vi "测量流程.vi"(11 "控制命令":T1(ring)) -> ()   [LabVIEW 2016, in "斯坦道氨氮V2.lvlib"]
panel:
  out "x-y":dbl
  out "当前时间":timestamp
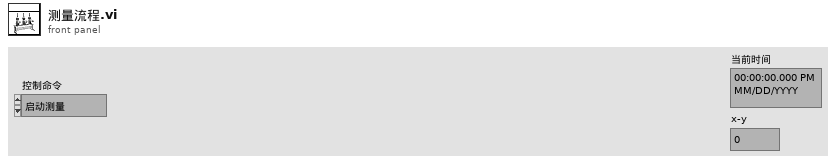
[diagram p1: front panel]
types:
  T1 = enum16{"启动测量", "标样核查", "零点核查", "跨度核查", "空白测试", "平行样测试", "加标回收", "空白校准", "标样校准", "初始化（清洗）", "停止测试", "仪器重启", "校时", "模式设置", "测量间隔设置"}
  T2 = cluster{"站号":u16, "量程切换":enum32{"H", "L", "AUTO"}, "控制命令":enum16{"启动测量", "标样核查", "零点核查", "跨度核查", "空白测试", "平行样测试", "加标回收", "空白校准", "标样校准", "初始化（清洗）", "停止测试", "仪器重启", "校时", "模式设置", "测量间隔设置"}, "模式设置":enum16{"待机", "连续模式", "周期模式", "定点模式", "受控模式", "手动模式"}, "测量间隔":u16}
  T3 = cluster{"时间标识":timestamp, "设备":string, "日志信息":string, "流程参数":string}
  T4 = enum16{"空闲", "水样测试", "标样核查", "零点核查", "跨度核查", "空白测试", "平行样测试", "加标回收", "空白校准", "标样校准", "初始化（清洗）"}
  T5 = cluster{"系统时间":timestamp, "工作状态":u16, "测量模式":enum16{"待机", "连续模式", "周期模式", "定点模式", "受控模式", "手动模式"}, "告警代码":u16, "故障代码":u16, "日志代码":u16, "软件版本":u16, "F0":sgl, "F1":sgl, "F2":sgl, "F3":sgl, "T":sgl, "H":sgl, "id":u16, "flowid":u16, "量程":u16, "总磷控温温度1":sgl, "营养盐控温温度2":sgl, "ADC":sgl}
  T6 = cluster{"水样测试量程模式":enum16{"H", "L", "AUTO"}, "空白核查量程模式":enum16{"H", "L", "AUTO"}, "跨度核查量程模式":enum16{"H", "L", "AUTO"}, "加标回收量程模式":enum16{"H", "L", "AUTO"}, "标样核查量程模式":enum16{"H", "L", "AUTO"}}
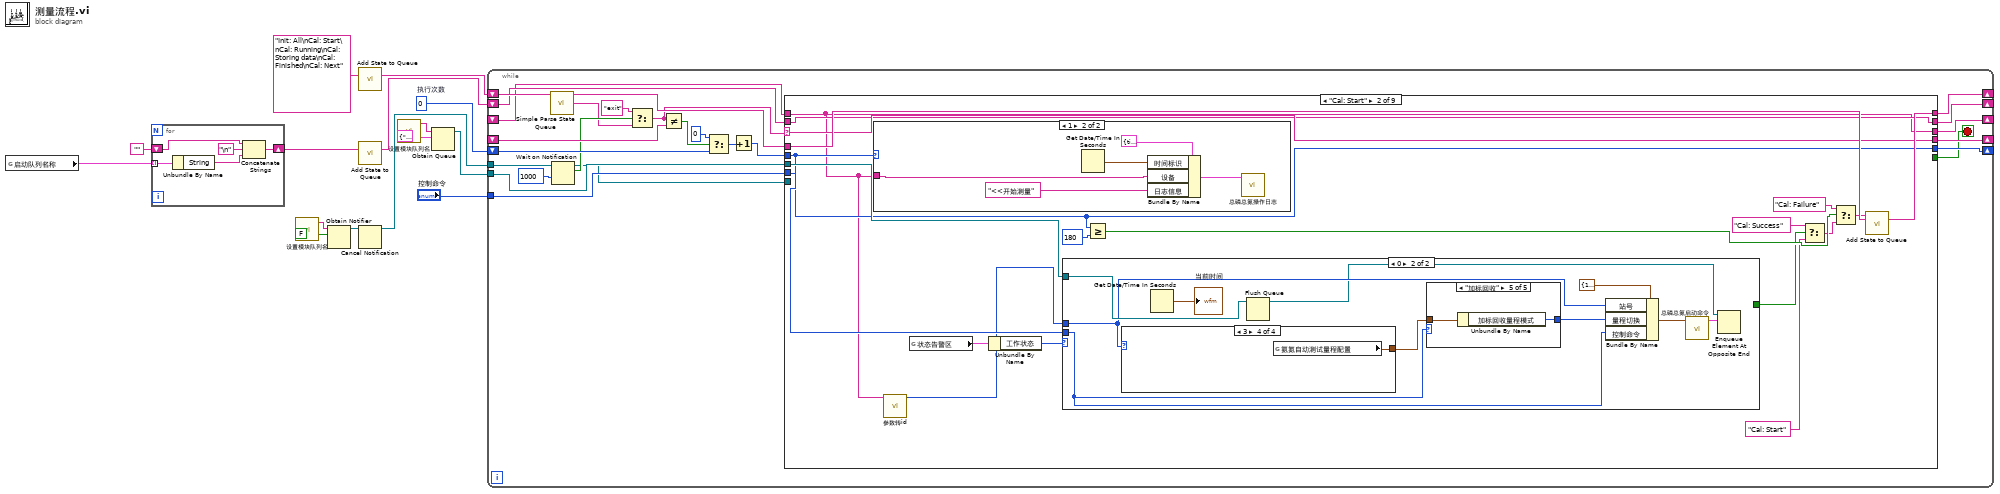
[diagram p0: block diagram]
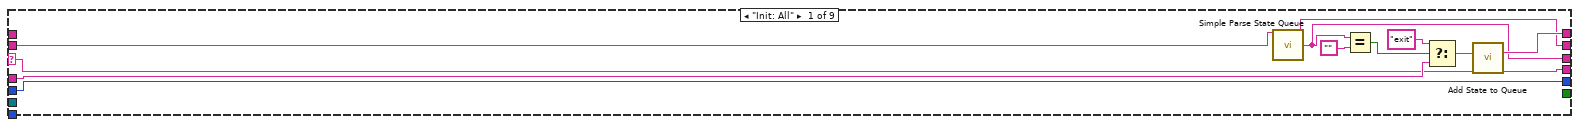
[diagram p2: hidden frame]
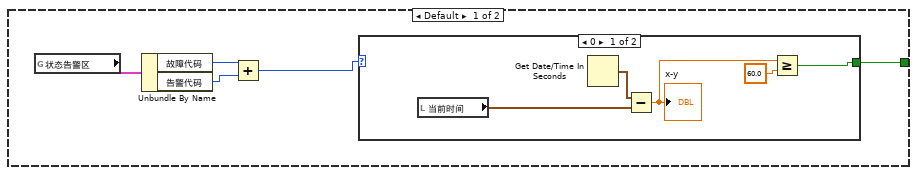
[diagram p3: hidden frame]
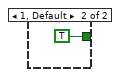
[diagram p4: hidden frame]
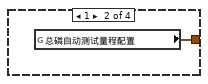
[diagram p6: hidden frame]
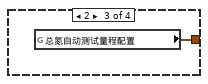
[diagram p7: hidden frame]
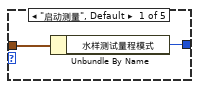
[diagram p8: hidden frame]
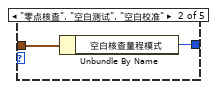
[diagram p9: hidden frame]
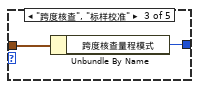
[diagram p10: hidden frame]
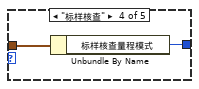
[diagram p11: hidden frame]
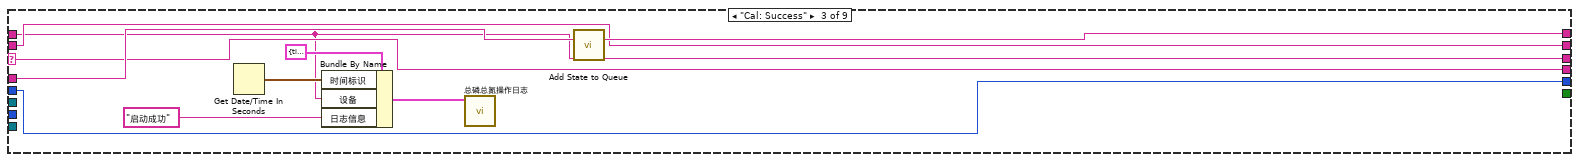
[diagram p13: hidden frame]
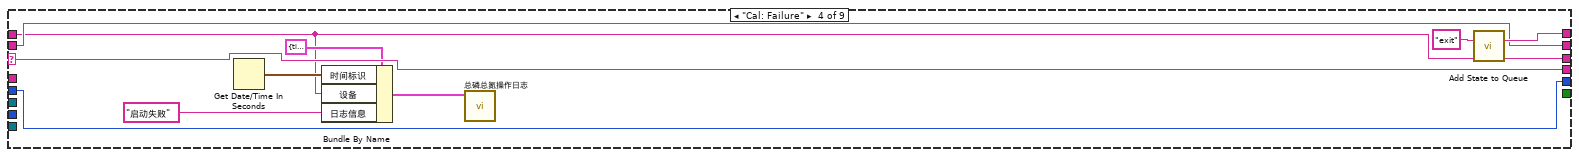
[diagram p14: hidden frame]
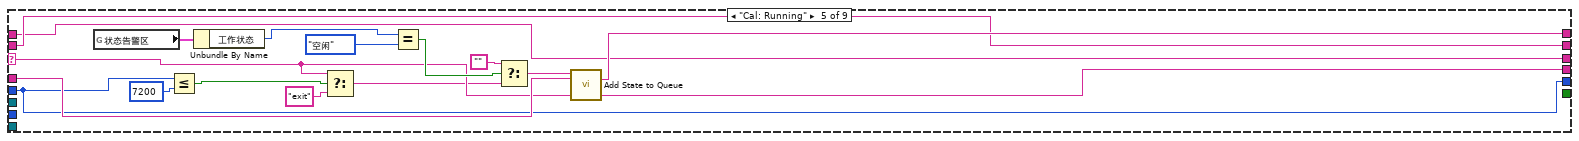
[diagram p15: hidden frame]
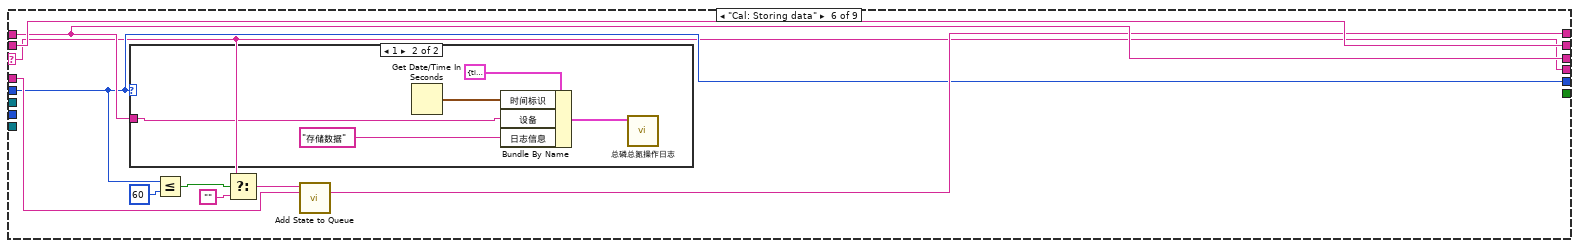
[diagram p16: hidden frame]
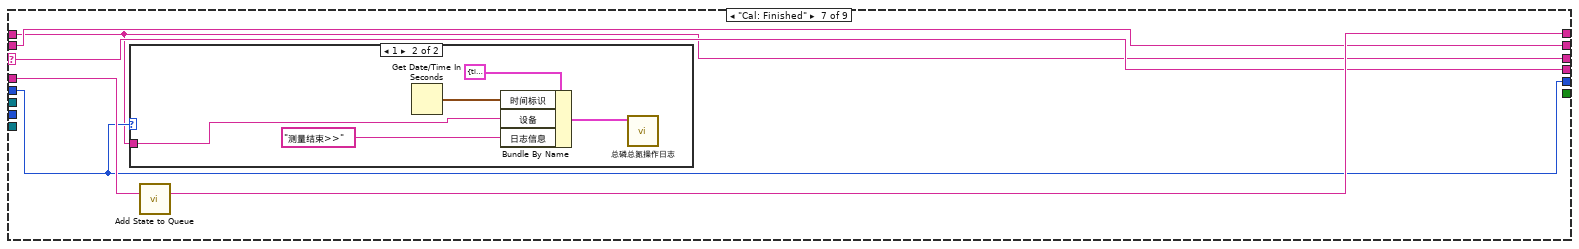
[diagram p18: hidden frame]
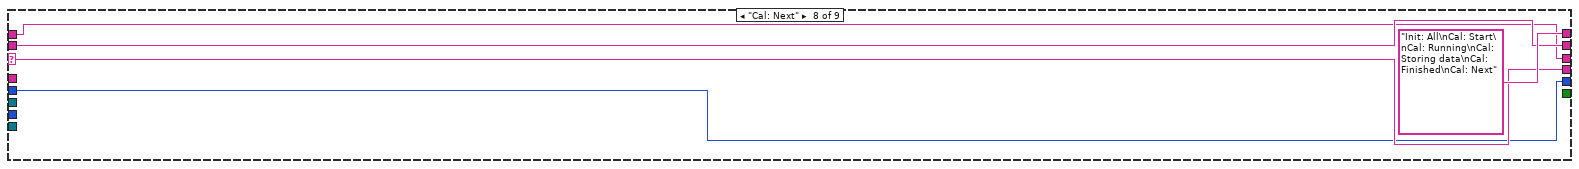
[diagram p20: hidden frame]
diagram:
  w9 = 0  # 执行次数
  n1 = global read "总磷总氮断电保存全局变量.vi" "启动队列名称"() -> (w1:cluster{"String":string, "Value":u16}[])
  n2 = for {
    shift-right: [w19] -> w2
    shift-left: "" -> [w20]
    tunnel: w1 -> [w18] mode=indexing
    n3 = Unbundle By Name(w18) -> ("String"=w17:string)
    n4 = Concatenate Strings(w20, "\n", w17) -> (w19:string)
  }
  n5 = call "设置模块队列名.vi"() -> ("Msg"=w6:string)  [unwired: 5 in]
  n6 = Obtain Notifier(name (unnamed)=w6, notification data type=FALSE) -> (notifier out=w14:refnum<notifier>)  [unwired: 2 in, 2 out]
  n7 = call "Add State to Queue.vi"("State(s) In (\"\")"="Init: All\nCal: Start\nCal: Running\nCal: Storing data\nCal: Finished\nCal: Next" ("State(s) In (\"\")")) -> ("States Out"=w12:string)  [unwired: 14 in]
  n8 = call "Add State to Queue.vi"("State(s) In (\"\")"=w2) -> ("States Out"=w7:string)  [unwired: 14 in]
  n9 = Cancel Notification(0:w14) -> (8:w4:refnum<notifier>)  [unwired: 1 in, 2 out]
  n10 = call "设置模块队列名.vi"() -> ("Msg"=w5:string)  [unwired: 5 in]
  n11 = Obtain Queue(name (unnamed)=w5, element data type=cluster{"命令":string, "data":variant} {"命令"="", "data"=variant}) -> (queue out=w10:refnum<queue>)  [unwired: 3 in, 2 out]
  n12 = while {
    tunnel: w10 -> [w43]
    shift-right: [w42] -> _
    shift-left: w12 -> [w45]
    shift-right: [w35] -> _
    shift-left: w9 -> [w38]
    shift-right: [w41] -> _
    shift-left: _ -> [w40]
    tunnel: "控制命令" -> [w33]
    shift-right: [w29] -> _
    shift-left: w7 -> [w31]
    shift-right: [w30] -> _
    shift-left: _ -> [w28]
    tunnel: w4 -> [w26]
    stop <- w32 stop-if-true
    n13 = call "Simple Parse State Queue.vi"("State Queue"=w45) -> ("Remain States"=w44:string, "Next State"=w23:string)  [unwired: 13 in]
    n14 = Wait on Notification(notifier=w26, timeout in ms (-1)=1000 ("超时毫秒(-1)")) -> (notifier out=w21:refnum<notifier>, notification=w25:bool)  [unwired: 2 in, 2 out]
    n15 = Select(t="exit", s=w25, f=w23) -> (s? t:f=w22:string)
    n16 = Not Equal?(x=w22, y=w40) -> (x != y?=w39:bool)
    n17 = Select(t=0, s=w39, f=w38) -> (s? t:f=w36:i32)
    n18 = Increment(x=w36) -> (x+1=w34:i32)
    n19 = case shown="\"Cal: Start\"" w22 {
      selector: w22 -> [w52 w73 w118 w133 w139 w153 w169 w180 w187]
      tunnel: w44 -> [w54 w75 w120 _ w150 w158 w171 _ w188]
      tunnel: w43 -> [_ w71 _ _ _ _ _ _ w183]
      tunnel: [w56 w74 w119 w134 w149 w157 w170 "Init: All\nCal: Start\nCal: Running\nCal: Storing data\nCal: Finished\nCal: Next" ("State(s) In (\"\")") w188] -> w42
      tunnel: [w52 w73 w118 w133 w139 w153 w169 w180 w187] -> w41
      tunnel: [w51 w69 w117 w132 w142 w156 w167 w179 w186] -> w35
      tunnel: w34 -> [w51 w69 w117 w132 w142 w156 w167 w179 w186]
      tunnel: w33 -> [_ w70 _ _ _ _ _ _ _]
      tunnel: [_ _ _ _ _ _ _ _ TRUE] -> w32
      tunnel: w31 -> [w50 w59 w116 w126 w136 w160 w168 w178 w185]
      tunnel: [w48 w58 w115 w125 w135 w159 w166 w177 w184] -> w30
      tunnel: [w49 w59 w116 w126 w136 w160 w168 w178 w185] -> w29
      tunnel: w28 -> [_ w58 w115 w125 w135 w159 w166 w177 w184]
      tunnel: w21 -> [_ _ _ _ _ _ _ _ w182]
      frame "Init: All" {
        n20 = call "Simple Parse State Queue.vi"("State Queue"=w50) -> ("Remain States"=w49:string, "Next State"=w48:string)  [unwired: 13 in]
        n21 = Equal?(x=w48, y="") -> (x = y?=w46:bool)
        n22 = Select(t="exit", s=w46, f=w54) -> (s? t:f=w53:string)
        n23 = call "Add State to Queue.vi"("State(s) In (\"\")"=w53) -> ("States Out"=w56:string)  [unwired: 14 in]
      }
      frame "Cal: Start" {
        n24 = case shown="1" w69 {
          tunnel: w58 -> [_ w110]
          frame 0, Default {
          }
          frame 1 {
            n25 = Get Date/Time In Seconds() -> (seconds since 1Jan1904=w114:timestamp)
            n26 = Bundle By Name(cluster=T3 {"时间标识"=timestamp(0 s since 1904-01-01), "设备"="", "日志信息"="", "流程参数"=""} ("data in"), "时间标识"=w114, "设备"=w110, "日志信息"="<<开始测量") -> (w113:T3)
            n27 = call "总磷总氮操作日志.vi"("data in"=w113) -> ()  [unwired: 10 in, 1 out]
          }
        }
        n28 = call "参数转id.vi"("table"=w58) -> ("id"=w57:u16)  [unwired: 10 in]
        n29 = global read "VAR总磷总氮全局变量.vi" "状态告警区"() -> (w72:T5)
        n30 = Unbundle By Name(w72) -> ("工作状态"=w60:u16)
        n31 = case shown="0" w60 {
          tunnel: w70 -> [_ w92]
          tunnel: w71 -> [_ w95]
          tunnel: [w80 _] -> w64
          tunnel: w57 -> [_ w90]
          frame Default {
            n32 = global read "VAR总磷总氮全局变量.vi" "状态告警区"() -> (w79:T5)
            n33 = Unbundle By Name(w79) -> ("故障代码"=w77:u16, "告警代码"=w78:u16)
            n34 = Add(x=w77, y=w78) -> (x+y=w76:u16)
            n35 = case shown="0" w76 {
              tunnel: [w81 TRUE] -> w80
              frame 0 {
                n36 = local read "当前时间"() -> (w85:timestamp)
                n37 = Get Date/Time In Seconds() -> (seconds since 1Jan1904=w84:timestamp)
                n38 = Subtract(x=w84, y=w85) -> (x-y=w83:dbl)
                "x-y" <- w83
                n39 = Greater Or Equal?(x=w83, y=60.0) -> (x >= y?=w81:bool)
              }
              frame 1, Default {
              }
            }
          }
          frame 0 {
            n40 = case shown="3" w90 {
              tunnel: [_ w97 w98 w99] -> w91
              frame 0, Default {
              }
              frame 1 {
                n41 = global read "总磷总氮断电保存全局变量.vi" "总磷自动测试量程配置"() -> (w97:T6)
              }
              frame 2 {
                n42 = global read "总磷总氮断电保存全局变量.vi" "总氮自动测试量程配置"() -> (w98:T6)
              }
              frame 3 {
                n43 = global read "总磷总氮断电保存全局变量.vi" "氨氮自动测试量程配置"() -> (w99:T6)
              }
            }
            n44 = Get Date/Time In Seconds() -> (seconds since 1Jan1904=→"当前时间":timestamp)
            n45 = Flush Queue(queue=w95) -> (queue out=w88:refnum<queue>)  [unwired: 1 in, 2 out]
            n46 = case shown="\"加标回收\"" w92 {
              tunnel: w91 -> [w101 w103 w105 w107 w109]
              tunnel: [w100 w102 w104 w106 w108] -> w96
              frame "启动测量", Default {
                n47 = Unbundle By Name(w101) -> ("水样测试量程模式"=w100:enum16{"H", "L", "AUTO"})
              }
              frame "零点核查", "空白测试", "空白校准" {
                n48 = Unbundle By Name(w103) -> ("空白核查量程模式"=w102:enum16{"H", "L", "AUTO"})
              }
              frame "跨度核查", "标样校准" {
                n49 = Unbundle By Name(w105) -> ("跨度核查量程模式"=w104:enum16{"H", "L", "AUTO"})
              }
              frame "标样核查" {
                n50 = Unbundle By Name(w107) -> ("标样核查量程模式"=w106:enum16{"H", "L", "AUTO"})
              }
              frame "加标回收" {
                n51 = Unbundle By Name(w109) -> ("加标回收量程模式"=w108:enum16{"H", "L", "AUTO"})
              }
            }
            n52 = Bundle By Name(cluster=T2 {"站号"=1, "量程切换"=enum."AUTO", "控制命令"=enum."启动测量", "模式设置"=enum."待机", "测量间隔"=0} ("参数"), "站号"=w90, "量程切换"=w96, "控制命令"=w92) -> (w93:T2)
            n53 = call "总磷总氮启动命令.vi"("参数"=w93) -> ("启动命令"=w89:cluster{"命令":string, "data":variant})  [unwired: 10 in]
            n54 = Enqueue Element At Opposite End(queue=w88, element=w89) -> ()  [unwired: 2 in, 3 out]
          }
        }
        n55 = Greater Or Equal?(x=w69, y=180) -> (x >= y?=w67:bool)
        n56 = Select(t="Cal: Success" ("State(s) In (\"\")"), s=w64, f="Cal: Start" ("State(s) In (\"\")")) -> (s? t:f=w62:string)
        n57 = Select(t="Cal: Failure" ("State(s) In (\"\")"), s=w67, f=w62) -> (s? t:f=w65:string)
        n58 = call "Add State to Queue.vi"("State(s) In Front (\"\")"=w65, "State(s) In (\"\")"=w75) -> ("States Out"=w74:string)  [unwired: 13 in]
      }
      frame "Cal: Success" {
        n59 = Get Date/Time In Seconds() -> (seconds since 1Jan1904=w123:timestamp)
        n60 = Bundle By Name(cluster=T3 {"时间标识"=timestamp(0 s since 1904-01-01), "设备"="", "日志信息"="", "流程参数"=""} ("data in"), "时间标识"=w123, "设备"=w115, "日志信息"="启动成功") -> (w122:T3)
        n61 = call "总磷总氮操作日志.vi"("data in"=w122) -> ()  [unwired: 10 in, 1 out]
        n62 = call "Add State to Queue.vi"("State(s) In (\"\")"=w120) -> ("States Out"=w119:string)  [unwired: 14 in]
      }
      frame "Cal: Failure" {
        n63 = Get Date/Time In Seconds() -> (seconds since 1Jan1904=w130:timestamp)
        n64 = Bundle By Name(cluster=T3 {"时间标识"=timestamp(0 s since 1904-01-01), "设备"="", "日志信息"="", "流程参数"=""} ("data in"), "时间标识"=w130, "设备"=w125, "日志信息"="启动失败") -> (w129:T3)
        n65 = call "总磷总氮操作日志.vi"("data in"=w129) -> ()  [unwired: 10 in, 1 out]
        n66 = call "Add State to Queue.vi"("State(s) In (\"\")"="exit" ("State(s) In (\"\")")) -> ("States Out"=w134:string)  [unwired: 14 in]
      }
      frame "Cal: Running" {
        n67 = global read "VAR总磷总氮全局变量.vi" "状态告警区"() -> (w146:T5)
        n68 = Less Or Equal?(x=w142, y=7200) -> (x <= y?=w140:bool)
        n69 = Unbundle By Name(w146) -> ("工作状态"=w147:u16)
        n70 = Select(t=w139, s=w140, f="exit") -> (s? t:f=w138:string)
        n71 = Equal?(x=w147, y=T4."空闲") -> (x = y?=w145:bool)
        n72 = Select(t="", s=w145, f=w138) -> (s? t:f=w143:string)
        n73 = call "Add State to Queue.vi"("State(s) In Front (\"\")"=w143, "State(s) In (\"\")"=w150) -> ("States Out"=w149:string)  [unwired: 13 in]
      }
      frame "Cal: Storing data" {
        n74 = case shown="1" w156 {
          tunnel: w159 -> [_ w161]
          frame 0, Default {
          }
          frame 1 {
            n75 = Get Date/Time In Seconds() -> (seconds since 1Jan1904=w165:timestamp)
            n76 = Bundle By Name(cluster=T3 {"时间标识"=timestamp(0 s since 1904-01-01), "设备"="", "日志信息"="", "流程参数"=""} ("data in"), "时间标识"=w165, "设备"=w161, "日志信息"="存储数据") -> (w164:T3)
            n77 = call "总磷总氮操作日志.vi"("data in"=w164) -> ()  [unwired: 10 in, 1 out]
          }
        }
        n78 = Less Or Equal?(x=w156, y=60) -> (x <= y?=w154:bool)
        n79 = Select(t=w153, s=w154, f="") -> (s? t:f=w151:string)
        n80 = call "Add State to Queue.vi"("State(s) In Front (\"\")"=w151, "State(s) In (\"\")"=w158) -> ("States Out"=w157:string)  [unwired: 13 in]
      }
      frame "Cal: Finished" {
        n81 = case shown="1" w167 {
          tunnel: w166 -> [_ w172]
          frame 0, Default {
          }
          frame 1 {
            n82 = Get Date/Time In Seconds() -> (seconds since 1Jan1904=w176:timestamp)
            n83 = Bundle By Name(cluster=T3 {"时间标识"=timestamp(0 s since 1904-01-01), "设备"="", "日志信息"="", "流程参数"=""} ("data in"), "时间标识"=w176, "设备"=w172, "日志信息"="测量结束>>") -> (w175:T3)
            n84 = call "总磷总氮操作日志.vi"("data in"=w175) -> ()  [unwired: 10 in, 1 out]
          }
        }
        n85 = call "Add State to Queue.vi"("State(s) In (\"\")"=w171) -> ("States Out"=w170:string)  [unwired: 14 in]
      }
      frame "Cal: Next" {
      }
      frame "exit", Default {
        n86 = Release Queue(queue=w183) -> ()  [unwired: 2 in, 3 out]
        n87 = Release Notifier(notifier=w182) -> ()  [unwired: 2 in, 3 out]
      }
    }
  }
